vi "Calculate LiDAR Measurement.vi"(10 "Old distance":dbl, 11 "unsigned byte array":u8[](array[numeric])) -> (3 "New distance":dbl)   [LabVIEW 2019]
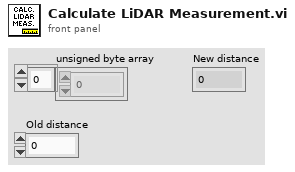
[diagram p1: front panel]
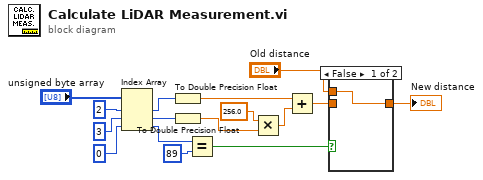
[diagram p0: block diagram]
diagram:
  n1 = Index Array(array="unsigned byte array", index #1=2 ("index"), index #2=3 ("index"), index #3=0 ("index")) -> (element #1=w7:u8, element #2=w6:u8, element #3=w13:u8)
  n2 = To Double Precision Float(number=w7) -> (double precision float=w11:dbl)
  n3 = To Double Precision Float(number=w6) -> (double precision float=w8:dbl)
  n4 = Equal?(x=w13, y=u8 89) -> (x = y?=w1:bool)
  n5 = Multiply(x=256.0, y=w8) -> (x*y=w10:dbl)
  n6 = Add(x=w11, y=w10) -> (x+y=w14:dbl)
  n7 = case shown="False" w1 {
    tunnel: w14 -> [_ w18]
    tunnel: [w17 w18] -> w15
    tunnel: "Old distance" -> [w17 _]
    frame False {
    }
    frame True {
    }
  }
  "New distance" <- w15
